vi "Transparent Image Overlay.vi"() -> ()   [LabVIEW 2011]
uses:
  <vilib>/picture/picture.llb/imagedata.ctl
  <vilib>/picture/picture.llb/Draw True-Color Pixmap.vi
panel:
  in  "image data":T1={"image type"=0, "image depth"=24, "image"=array[49050 elements], "mask"=[], "colors"=[], "Rectangle"={"left"=0, "top"=0, "right"=109, "bottom"=150}} caption="图像数据"
  in  "Circle Overlays":T2(array[cluster])=[{"pixel center"={"horizontal"=50, "vertical"=50}, "radius"=30, "circle color"=16711680}, {"pixel center"={"horizontal"=20, "vertical"=20}, "radius"=30, "circle color"=327900}, {"pixel center"={"horizontal"=100, "vertical"=100}, "radius"=30, "circle color"=1985280}]
  in  "Transparency Factor":dbl(slide)=0.5757575757575758 min=0.0 max=1.0 step=0.05 scale=0.0..1.0
  out "Original Image":picture
  out "Overlay":picture
  out "Final Image":picture
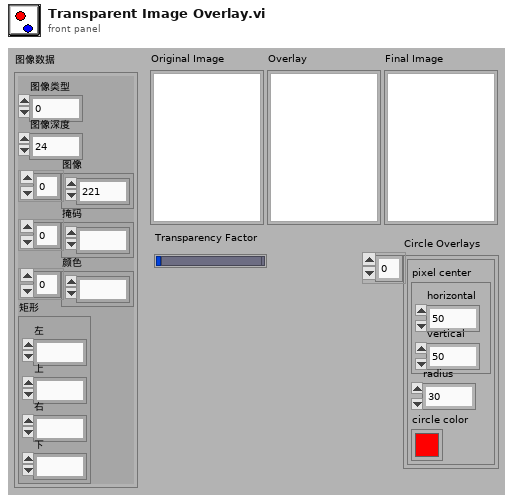
[diagram p1: front panel]
types:
  T1 = typedef "imagedata.ctl" = cluster{"image type":i32, "image depth":i32, "image":u8[], "mask":u8[], "colors":u32[], "Rectangle":cluster{"left":i16, "top":i16, "right":i16, "bottom":i16}}
  T2 = cluster{"pixel center":cluster{"horizontal":i16, "vertical":i16}, "radius":i16, "circle color":u32}[]
  T3 = cluster{"left":i16, "top":i16, "right":i16, "bottom":i16}
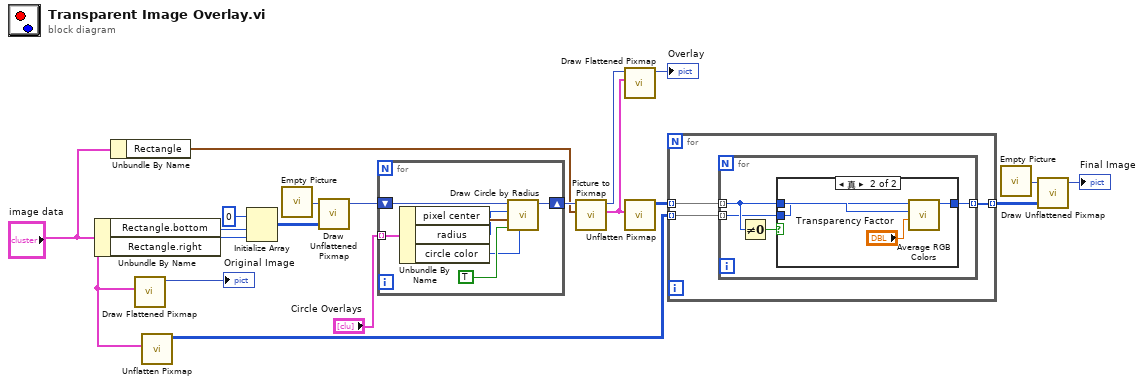
[diagram p0: block diagram]
diagram:
  n1 = Unbundle By Name("image data") -> ("Rectangle.bottom"=w17:i16, "Rectangle.right"=w16:i16)
  n2 = Unbundle By Name("image data") -> ("Rectangle"=w1:T3)
  n3 = call <vilib>:"Draw Flattened Pixmap.vi"("image data"="image data") -> ("new picture"=→"Original Image":picture)  [unwired: 8 in]
  n4 = call <vilib>:"Unflatten Pixmap.vi"("image data"="image data") -> ("24-bit pixmap"=w14:u32[][])  [unwired: 4 in, 6 out]
  n5 = Initialize Array(u32 0, w17, w16) -> (w15:u32[][])
  n6 = call "Empty Picture"() -> ("empty picture"=w19:picture)
  n7 = call-poly <vilib>:"Draw Unflattened Pixmap.vi"("picture"=w19, "data (RGB format)"=w15) -> ("new picture"=w8:picture)  [unwired: 7 in]
  n8 = for {
    shift-right: [w24] -> w6
    shift-left: w8 -> [w25]
    tunnel: "Circle Overlays" -> [w23] mode=indexing
    n9 = Unbundle By Name(w23) -> ("pixel center"=w22:cluster{"horizontal":i16, "vertical":i16}, "radius"=w21:i16, "circle color"=w20:u32)
    n10 = call <vilib>:"Draw Circle by Radius.vi"("color(black)"=w20, "fill?(F)"=TRUE, "pixel center"=w22, "radius"=w21, "picture"=w25) -> ("new picture"=w24:picture)  [unwired: 6 in]
  }
  n11 = call <vilib>:"Picture to Pixmap.vi"("rect"=w1, "picture"=w6) -> ("image data"=w9:T1, "new picture"=w4:picture)  [unwired: 8 in]
  n12 = call <vilib>:"Draw Flattened Pixmap.vi"("image data"=w9, "picture"=w4) -> ("new picture"=→"Overlay":picture)  [unwired: 7 in]
  n13 = call <vilib>:"Unflatten Pixmap.vi"("image data"=w9) -> ("24-bit pixmap"=w11:u32[][])  [unwired: 4 in, 6 out]
  n14 = for {
    tunnel: w14 -> [w28] mode=indexing
    tunnel: w11 -> [w29] mode=indexing
    tunnel: [w27] -> w10 mode=indexing
    n15 = for {
      tunnel: w29 -> [w32] mode=indexing
      tunnel: w28 -> [w31] mode=indexing
      tunnel: [w30] -> w27 mode=indexing
      n16 = Not Equal To 0?(x=w32) -> (x != 0?=w33:bool)
      n17 = case shown="真" w33 {
        tunnel: w32 -> [_ w38]
        tunnel: w31 -> [w34 w37]
        tunnel: [w34 w36] -> w30
        frame False {
        }
        frame True {
          n18 = call "Average RGB Colors.vi"("Transparency Factor"="Transparency Factor", "x"=w38, "y"=w37) -> ("result"=w36:u32)  [unwired: 8 in]
        }
      }
    }
  }
  n19 = call "Empty Picture"() -> ("empty picture"=w12:picture)
  n20 = call-poly <vilib>:"Draw Unflattened Pixmap.vi"("picture"=w12, "data (RGB format)"=w10) -> ("new picture"=→"Final Image":picture)  [unwired: 7 in]
